vi "auton drive.vi"   [LabVIEW 2013]
types:
  T1 = typedef "WPI_EncoderDevRef.ctl" = cluster{"DevStatus":errorcluster, "EncoderIndex":T2, "CounterIndex":T3, "DistancePerCount":dbl, "Decoding Type":T4}
  T2 = typedef "FPGA_EncoderIdx.ctl" = enum8{"Enc 0", "Enc 1", "Enc 2", "Enc 3", "Invalid"}
  T3 = typedef "FPGA_CounterCtrSystemIndex.ctl" = enum8{"Ctr 0", "Ctr 1", "Ctr 2", "Ctr 3", "Ctr 4", "Ctr 5", "Ctr 6", "Ctr 7", "Invalid"}
  T4 = typedef "WPI_EncoderType.ctl" = enum16{"1x", "2x", "4x"}
  T5 = typedef "WPI_GyroDevRef.ctl" = cluster{"DevStatus":errorcluster, "Analog Module":T6, "Analog Channel":T7, "Offset":dbl, "Gain (VoltsPerDegree/Second)":dbl}
  T6 = typedef "FPGA_TypedefAnalogModule.ctl" = enum16{"Analog Module 1", "Analog Module 2"}
  T7 = typedef "FPGA_AIChannel.ctl" = enum8{"AI 1", "AI 2", "AI 3", "AI 4", "AI 5", "AI 6", "AI 7", "AI 8", "Invalid"}
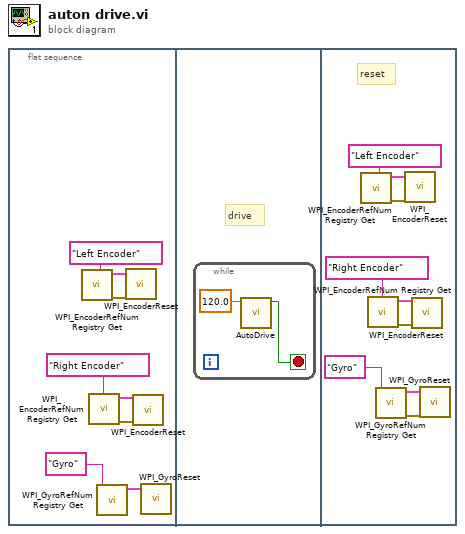
[diagram p0: block diagram]
diagram:
  n1 = flat-sequence {
    frame #0 {
      n2 = call <vilib>:"WPI_EncoderRefNum Registry Get.vi"("refnum name"="Left Encoder") -> ("error out"=w8:errorcluster, "EncoderDevRef"=w7:T1)  [unwired: 9 in]
      n3 = call <vilib>:"WPI_EncoderRefNum Registry Get.vi"("refnum name"="Right Encoder") -> ("error out"=w6:errorcluster, "EncoderDevRef"=w5:T1)  [unwired: 9 in]
      n4 = call <vilib>:"WPI_GyroRefNum Registry Get.vi"("refnum name"="Gyro") -> ("GyroDevRef"=w1:T5)  [unwired: 9 in, 1 out]
      n5 = call <vilib>:"WPI_EncoderReset.vi"("error in (no error)"=w8, "EncoderDevRef"=w7) -> ()  [unwired: 8 in, 2 out]
      n6 = call <vilib>:"WPI_EncoderReset.vi"("error in (no error)"=w6, "EncoderDevRef"=w5) -> ()  [unwired: 8 in, 2 out]
      n7 = call <vilib>:"WPI_GyroReset.vi"("GyroDevRef"=w1) -> ()  [unwired: 9 in, 2 out]
    }
    frame #1 {
      # "drive"
      n8 = while {
        stop <- w9 stop-if-true
        n9 = call "AutoDrive.vi"("Target"=120.0) -> ("Reached Target"=w9:bool)  [unwired: 10 in]
      }
    }
    frame #2 {
      # "reset"
      n10 = call <vilib>:"WPI_EncoderRefNum Registry Get.vi"("refnum name"="Left Encoder") -> ("error out"=w11:errorcluster, "EncoderDevRef"=w12:T1)  [unwired: 9 in]
      n11 = call <vilib>:"WPI_EncoderRefNum Registry Get.vi"("refnum name"="Right Encoder") -> ("error out"=w13:errorcluster, "EncoderDevRef"=w14:T1)  [unwired: 9 in]
      n12 = call <vilib>:"WPI_GyroRefNum Registry Get.vi"("refnum name"="Gyro") -> ("error out"=w18:errorcluster, "GyroDevRef"=w19:T5)  [unwired: 9 in]
      n13 = call <vilib>:"WPI_EncoderReset.vi"("error in (no error)"=w11, "EncoderDevRef"=w12) -> ()  [unwired: 8 in, 2 out]
      n14 = call <vilib>:"WPI_EncoderReset.vi"("error in (no error)"=w13, "EncoderDevRef"=w14) -> ()  [unwired: 8 in, 2 out]
      n15 = call <vilib>:"WPI_GyroReset.vi"("error in (no error)"=w18, "GyroDevRef"=w19) -> ()  [unwired: 8 in, 2 out]
    }
  }
